vi "25_P-GPIB-LockIn510.vi"(2 "Tipo":u16(ring)=1 items=["LockIn", "LockIn-DMM"], 3 "Lecturas":i32=1, 4 "P-DMM":string="16", 5 "P-LockIn":string="20") -> (0 "DMM":dbl, 1 "LockIn":dbl)   [LabVIEW 2016]
uses:
  <vilib>/Utility/error.llb/DialogType.ctl
panel:
  out "Cont-C":i32=50
  out "Cont-B":i32=50
  out "Cont-A":i32=50
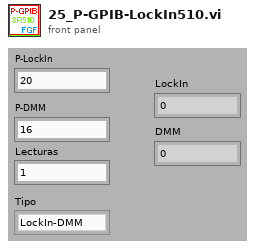
[diagram p1: front panel]
types:
  T1 = typedef "DialogType.ctl" = u16
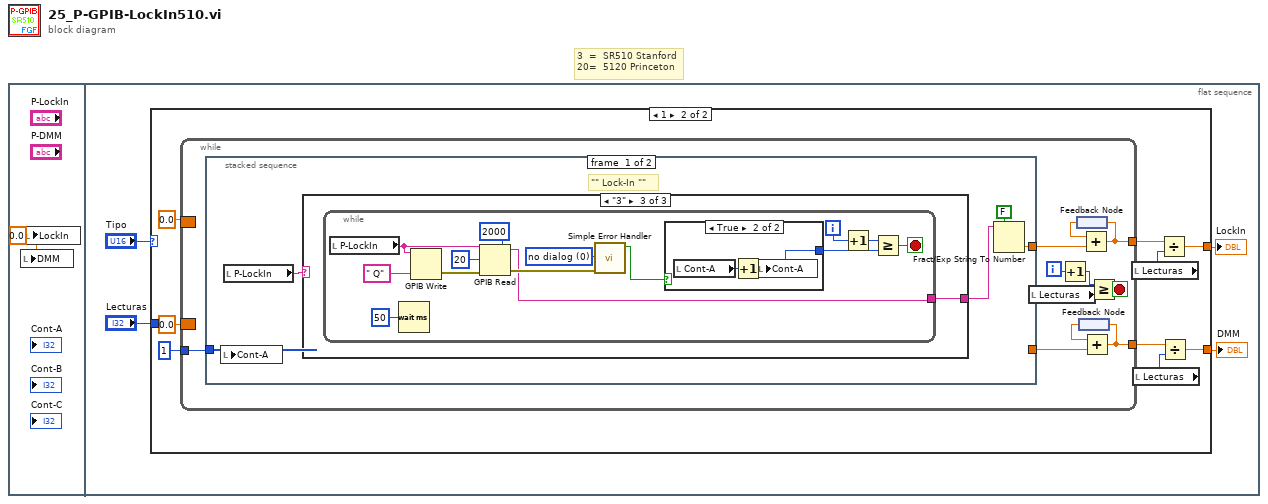
[diagram p0: block diagram]
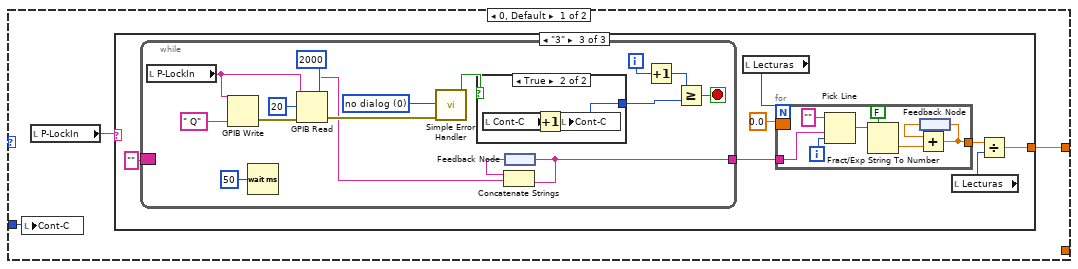
[diagram p2: hidden frame]
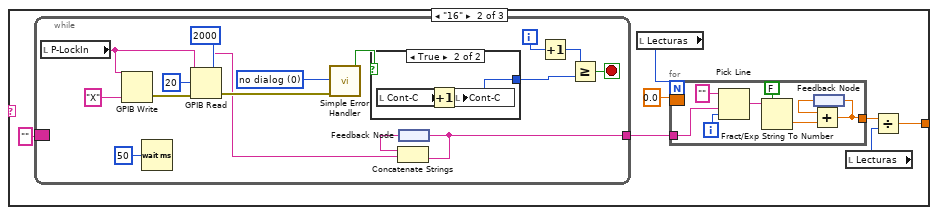
[diagram p4: hidden frame]
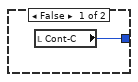
[diagram p5: hidden frame]
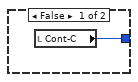
[diagram p6: hidden frame]
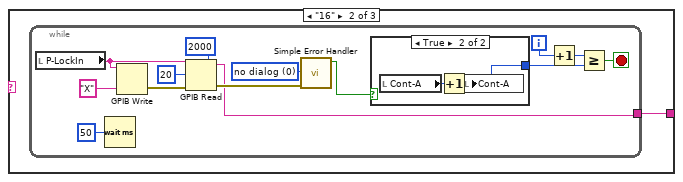
[diagram p8: hidden frame]
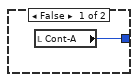
[diagram p9: hidden frame]
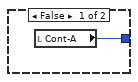
[diagram p10: hidden frame]
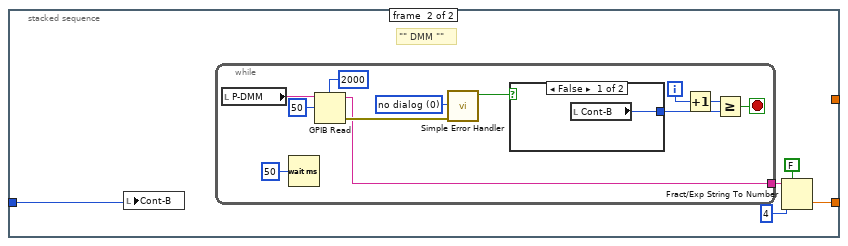
[diagram p11: hidden frame]
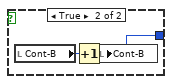
[diagram p12: hidden frame]
diagram:
  # "3  =  SR510 Stanford\n20=  5120 Princeton"
  n1 = flat-sequence {
    frame #0 {
      w1 = 0.0 ("LockIn")
      n2 = local write "DMM"(w1) -> ()
      n3 = local write "LockIn"(w1) -> ()
    }
    frame #1 {
      n4 = case shown="1" "Tipo" {
        tunnel: [w8 w80] -> w5
        tunnel: [_ w79] -> w4
        tunnel: "Lecturas" -> [w7 _]
        frame 0, Default {
          n5 = local write "Cont-C"(w7) -> ()
          n6 = local read "P-LockIn"() -> (w6:string)
          n7 = case shown="\"3\"" w6 {
            tunnel: [_ w9 w43] -> w8
            frame "False", Default {
            }
            frame "16" {
              n8 = while {
                border: "" -> [_]
                tunnel: [w27] -> w15
                i -> [w39]
                stop <- w36 stop-if-true
                w31 = T1 0 items=["no dialog", "OK message", "continue or stop message", "OK message + warnings", "continue/stop + warnings"] ("type of dialog (OK msg:1)")
                n9 = local read "P-LockIn"() -> (w28:string)
                n10 = GPIB Write(0:w28, 1:"X" ("Write")) -> (6:w33:errorcluster)  [unwired: 3 in, 1 out]
                n11 = Wait (ms)(milliseconds to wait=u32 50) -> ()  [unwired: 1 out]
                n12 = GPIB Read(0:w28, 1:20 ("# Bytes to Read"), 3:w33, 4:2000 ("timeout ms (488.2 global)")) -> (5:w25:string, 7:w30:errorcluster)  [unwired: 1 in, 1 out]
                n13 = call <vilib>:"Simple Error Handler.vi"("type of dialog (OK msg:1)"=w31, "error in (no error)"=w30) -> ("error?"=w26:bool)  [unwired: 3 in, 4 out]
                n14 = case shown="True" w26 {
                  tunnel: [w40 w41] -> w38
                  frame False {
                    n15 = local read "Cont-C"() -> (w40:i32)
                  }
                  frame True {
                    n16 = local read "Cont-C"() -> (w42:i32)
                    n17 = Increment(x=w42) -> (x+1=w41:i32)
                    n18 = local write "Cont-C"(w41) -> ()
                  }
                }
                n19 = feedback #1() -> (w29:string)
                n20 = Concatenate Strings(w29, w25) -> (w27:string)
                n21 = feedback-in #1(w27) -> ()
                n22 = Increment(x=w39) -> (x+1=w37:i32)
                n23 = Greater Or Equal?(x=w37, y=w38) -> (x >= y?=w36:bool)
              }
              n24 = local read "Lecturas"() -> (w13:i32)
              n25 = for {
                N: w13 -> [_]
                border: 0.0 -> [_]
                tunnel: [w19] -> w12
                tunnel: w15 -> [w18]
                i -> [w23]
                n26 = Pick Line(string ("")="", multi-line string=w18, line index=w23) -> (output string=w17:string)
                n27 = Fract/Exp String To Number(use system decimal point (T)=FALSE, string=w17) -> (number=w16:dbl)  [unwired: 2 in, 1 out]
                n28 = feedback #2() -> (w20:dbl)
                n29 = Add(x=w20, y=w16) -> (x+y=w19:dbl)
                n30 = feedback-in #2(w19) -> ()
              }
              n31 = local read "Lecturas"() -> (w11:i32)
              n32 = Divide(x=w12, y=w11) -> (x/y=w9:dbl)
            }
            frame "3" {
              n33 = while {
                border: "" -> [_]
                tunnel: [w61] -> w49
                i -> [w73]
                stop <- w70 stop-if-true
                w65 = T1 0 items=["no dialog", "OK message", "continue or stop message", "OK message + warnings", "continue/stop + warnings"] ("type of dialog (OK msg:1)")
                n34 = local read "P-LockIn"() -> (w62:string)
                n35 = GPIB Write(0:w62, 1:" Q" ("Write")) -> (6:w67:errorcluster)  [unwired: 3 in, 1 out]
                n36 = Wait (ms)(milliseconds to wait=u32 50) -> ()  [unwired: 1 out]
                n37 = GPIB Read(0:w62, 1:20 ("# Bytes to Read"), 3:w67, 4:2000 ("timeout ms (488.2 global)")) -> (5:w59:string, 7:w64:errorcluster)  [unwired: 1 in, 1 out]
                n38 = call <vilib>:"Simple Error Handler.vi"("type of dialog (OK msg:1)"=w65, "error in (no error)"=w64) -> ("error?"=w60:bool)  [unwired: 3 in, 4 out]
                n39 = case shown="True" w60 {
                  tunnel: [w74 w75] -> w72
                  frame False {
                    n40 = local read "Cont-C"() -> (w74:i32)
                  }
                  frame True {
                    n41 = local read "Cont-C"() -> (w76:i32)
                    n42 = Increment(x=w76) -> (x+1=w75:i32)
                    n43 = local write "Cont-C"(w75) -> ()
                  }
                }
                n44 = feedback #3() -> (w63:string)
                n45 = Concatenate Strings(w63, w59) -> (w61:string)
                n46 = feedback-in #3(w61) -> ()
                n47 = Increment(x=w73) -> (x+1=w71:i32)
                n48 = Greater Or Equal?(x=w71, y=w72) -> (x >= y?=w70:bool)
              }
              n49 = local read "Lecturas"() -> (w47:i32)
              n50 = for {
                N: w47 -> [_]
                border: 0.0 -> [_]
                tunnel: [w53] -> w46
                tunnel: w49 -> [w52]
                i -> [w57]
                n51 = Pick Line(string ("")="", multi-line string=w52, line index=w57) -> (output string=w51:string)
                n52 = Fract/Exp String To Number(use system decimal point (T)=FALSE, string=w51) -> (number=w50:dbl)  [unwired: 2 in, 1 out]
                n53 = feedback #4() -> (w54:dbl)
                n54 = Add(x=w54, y=w50) -> (x+y=w53:dbl)
                n55 = feedback-in #4(w53) -> ()
              }
              n56 = local read "Lecturas"() -> (w45:i32)
              n57 = Divide(x=w46, y=w45) -> (x/y=w43:dbl)
            }
          }
        }
        frame 1 {
          n58 = while {
            border: 0.0 -> [_]
            tunnel: 1 ("Cont-A") -> [w93]
            border: 0.0 -> [_]
            tunnel: [w87] -> w81
            tunnel: [w90] -> w78
            i -> [w94]
            stop <- w95 stop-if-true
            n59 = stacked-sequence {
              tunnel: w93 -> [w98 w139]
              tunnel: [w99 _] -> w86
              tunnel: [_ w140] -> w91
              frame #0 {
                # "\"\" Lock-In \"\""
                n60 = local write "Cont-A"(w98) -> ()
                n61 = local read "P-LockIn"() -> (w97:string)
                n62 = case shown="\"3\"" w97 {
                  tunnel: [_ w102 w120] -> w100
                  frame "False", Default {
                  }
                  frame "16" {
                    n63 = while {
                      tunnel: [w104] -> w102
                      i -> [w116]
                      stop <- w113 stop-if-true
                      w110 = T1 0 items=["no dialog", "OK message", "continue or stop message", "OK message + warnings", "continue/stop + warnings"] ("type of dialog (OK msg:1)")
                      n64 = local read "P-LockIn"() -> (w112:string)
                      n65 = Wait (ms)(milliseconds to wait=u32 50) -> ()  [unwired: 1 out]
                      n66 = GPIB Write(0:w112, 1:"X" ("Write")) -> (6:w108:errorcluster)  [unwired: 3 in, 1 out]
                      n67 = GPIB Read(0:w112, 1:20 ("# Bytes to Read"), 3:w108, 4:2000 ("timeout ms (488.2 global)")) -> (5:w104:string, 7:w111:errorcluster)  [unwired: 1 in, 1 out]
                      n68 = call <vilib>:"Simple Error Handler.vi"("type of dialog (OK msg:1)"=w110, "error in (no error)"=w111) -> ("error?"=w105:bool)  [unwired: 3 in, 4 out]
                      n69 = case shown="True" w105 {
                        tunnel: [w117 w118] -> w115
                        frame False {
                          n70 = local read "Cont-A"() -> (w117:i32)
                        }
                        frame True {
                          n71 = local read "Cont-A"() -> (w119:i32)
                          n72 = Increment(x=w119) -> (x+1=w118:i32)
                          n73 = local write "Cont-A"(w118) -> ()
                        }
                      }
                      n74 = Increment(x=w116) -> (x+1=w114:i32)
                      n75 = Greater Or Equal?(x=w114, y=w115) -> (x >= y?=w113:bool)
                    }
                  }
                  frame "3" {
                    n76 = while {
                      tunnel: [w122] -> w120
                      i -> [w134]
                      stop <- w131 stop-if-true
                      w128 = T1 0 items=["no dialog", "OK message", "continue or stop message", "OK message + warnings", "continue/stop + warnings"] ("type of dialog (OK msg:1)")
                      n77 = local read "P-LockIn"() -> (w130:string)
                      n78 = Wait (ms)(milliseconds to wait=u32 50) -> ()  [unwired: 1 out]
                      n79 = GPIB Write(0:w130, 1:" Q" ("Write")) -> (6:w126:errorcluster)  [unwired: 3 in, 1 out]
                      n80 = GPIB Read(0:w130, 1:20 ("# Bytes to Read"), 3:w126, 4:2000 ("timeout ms (488.2 global)")) -> (5:w122:string, 7:w129:errorcluster)  [unwired: 1 in, 1 out]
                      n81 = call <vilib>:"Simple Error Handler.vi"("type of dialog (OK msg:1)"=w128, "error in (no error)"=w129) -> ("error?"=w123:bool)  [unwired: 3 in, 4 out]
                      n82 = case shown="True" w123 {
                        tunnel: [w135 w136] -> w133
                        frame False {
                          n83 = local read "Cont-A"() -> (w135:i32)
                        }
                        frame True {
                          n84 = local read "Cont-A"() -> (w137:i32)
                          n85 = Increment(x=w137) -> (x+1=w136:i32)
                          n86 = local write "Cont-A"(w136) -> ()
                        }
                      }
                      n87 = Increment(x=w134) -> (x+1=w132:i32)
                      n88 = Greater Or Equal?(x=w132, y=w133) -> (x >= y?=w131:bool)
                    }
                  }
                }
                n89 = Fract/Exp String To Number(use system decimal point (T)=FALSE, string=w100) -> (number=w99:dbl)  [unwired: 2 in, 1 out]
              }
              frame #1 {
                # "\"\" DMM \"\""
                n90 = local write "Cont-B"(w139) -> ()
                n91 = while {
                  tunnel: [w144] -> w141
                  i -> [w154]
                  stop <- w151 stop-if-true
                  w148 = T1 0 items=["no dialog", "OK message", "continue or stop message", "OK message + warnings", "continue/stop + warnings"] ("type of dialog (OK msg:1)")
                  n92 = local read "P-DMM"() -> (w146:string)
                  n93 = Wait (ms)(milliseconds to wait=u32 50) -> ()  [unwired: 1 out]
                  n94 = GPIB Read(0:w146, 1:50 ("# Bytes to Read"), 4:2000 ("timeout ms (488.2 global)")) -> (5:w144:string, 7:w147:errorcluster)  [unwired: 2 in, 1 out]
                  n95 = call <vilib>:"Simple Error Handler.vi"("type of dialog (OK msg:1)"=w148, "error in (no error)"=w147) -> ("error?"=w145:bool)  [unwired: 3 in, 4 out]
                  n96 = case shown="False" w145 {
                    tunnel: [w155 w156] -> w153
                    frame False {
                      n97 = local read "Cont-B"() -> (w155:i32)
                    }
                    frame True {
                      n98 = local read "Cont-B"() -> (w157:i32)
                      n99 = Increment(x=w157) -> (x+1=w156:i32)
                      n100 = local write "Cont-B"(w156) -> ()
                    }
                  }
                  n101 = Increment(x=w154) -> (x+1=w152:i32)
                  n102 = Greater Or Equal?(x=w152, y=w153) -> (x >= y?=w151:bool)
                }
                n103 = Fract/Exp String To Number(use system decimal point (T)=FALSE, string=w141, offset=4) -> (number=w140:dbl)  [unwired: 1 in, 1 out]
              }
            }
            n104 = local read "Lecturas"() -> (w89:i32)
            n105 = Increment(x=w94) -> (x+1=w88:i32)
            n106 = feedback #5() -> (w96:dbl)
            n107 = feedback #6() -> (w92:dbl)
            n108 = Add(x=w96, y=w86) -> (x+y=w87:dbl)
            n109 = feedback-in #5(w87) -> ()
            n110 = Add(x=w92, y=w91) -> (x+y=w90:dbl)
            n111 = feedback-in #6(w90) -> ()
            n112 = Greater Or Equal?(x=w88, y=w89) -> (x >= y?=w95:bool)
          }
          n113 = local read "Lecturas"() -> (w83:i32)
          n114 = local read "Lecturas"() -> (w82:i32)
          n115 = Divide(x=w81, y=w83) -> (x/y=w80:dbl)
          n116 = Divide(x=w78, y=w82) -> (x/y=w79:dbl)
        }
      }
      "LockIn" <- w5
      "DMM" <- w4
    }
  }
